vi "nRF24 communication.vi"(8 "error in (no error)":errorcluster) -> (0 "error out":errorcluster)   [LabVIEW 2016]
uses:
  Typedef/Remote Control Cluster.ctl
  Typedef/INS Data.ctl
  Shared resoruces/gear.vi
  Shared resoruces/ODrive State and Info.vi
  Shared resoruces/Navigation Variables.vi
  Shared resoruces/Shared resources RT.lvlib
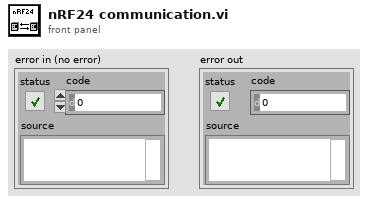
[diagram p1: front panel]
types:
  T1 = typedef "Semaphore RefNum" = refnum<k1>
  T2 = typedef "INS Data.ctl" = cluster{"Yaw":sgl, "Pitch":sgl, "Roll":sgl, "Lat":dbl, "Long":dbl, "Alt":dbl, "North":dbl, "East":dbl, "Down":dbl, "PosU":dbl, "VelU":dbl}
  T3 = typedef "Remote Control Cluster.ctl" = cluster{"Pot1":u16, "Pot2":u16, "Pot3":u16, "Pot4":u16, "Switch1":cluster{"L":bool, "H":bool}, "Switch2":cluster{"L":bool, "H":bool}, "Switch3":cluster{"L":bool, "H":bool}}
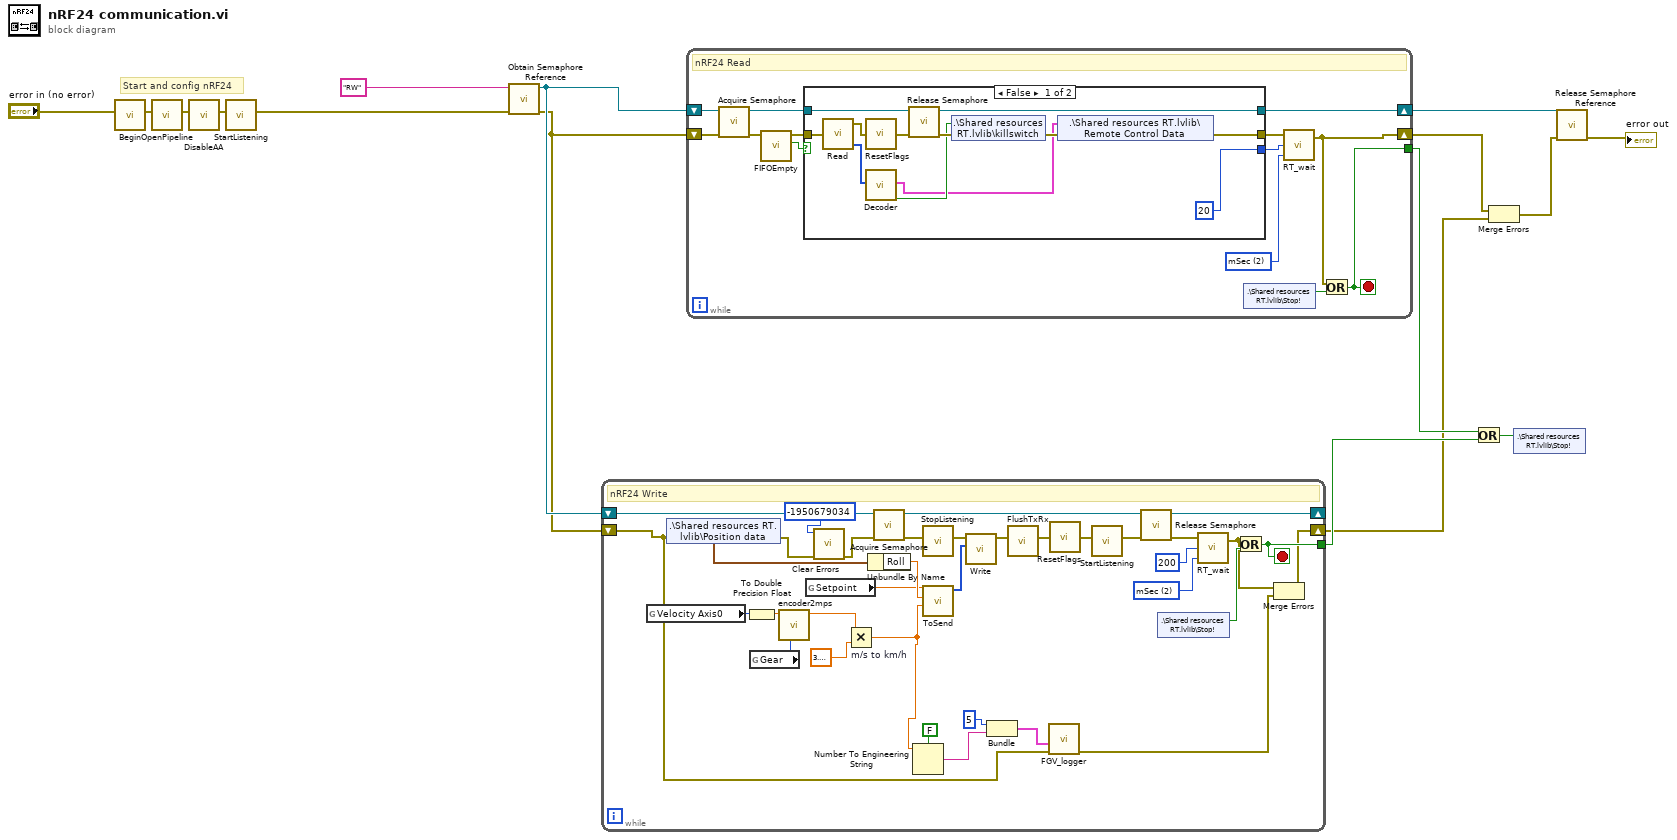
[diagram p0: block diagram]
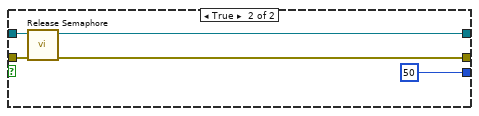
[diagram p2: hidden frame]
diagram:
  # "Start and config nRF24"
  n1 = call "Begin.vi"("error in (no error)"="error in (no error)") -> ("error out"=w2:errorcluster)  [unwired: 10 in]
  n2 = call "OpenPipeline.vi"("error in (no error)"=w2) -> ("error out"=w3:errorcluster)  [unwired: 10 in]
  n3 = call "DisableAA.vi"("error in (no error)"=w3) -> ("error out"=w4:errorcluster)  [unwired: 10 in]
  n4 = call "StartListening.vi"("error in (no error)"=w4) -> ("error out"=w5:errorcluster)  [unwired: 10 in]
  n5 = call <vilib>:"Obtain Semaphore Reference.vi"("error in (no error)"=w5, "name (unnamed)"="RW") -> ("error out"=w7:errorcluster, "semaphore"=w8:T1)  [unwired: 3 in, 1 out]
  n6 = while {
    shift-right: [w45] -> _
    shift-left: w8 -> [w51]
    shift-right: [w28] -> w10
    shift-left: w7 -> [w30]
    tunnel: [w36] -> w14
    stop <- w36 stop-if-true
    w42 = u16 2 items=["Ticks", "uSec", "mSec"] ("Counter Units")
    # "nRF24 Write"
    n7 = global read "ODrive State and Info.vi" "Velocity Axis0"() -> (w19:i16)
    n8 = shared-variable ".\\Shared resources RT.lvlib\\Position data"(error in=w30) -> (w35:T2, error out=w26:errorcluster)
    n9 = To Double Precision Float(number=w19) -> (double precision float=w18:dbl)
    n10 = global read "gear.vi" "Gear"() -> (w20:enum16{"7", "6", "5", "4", "3", "2", "1"})
    n11 = call "encoder2mps.vi"("Gear"=w20, "encoderSpeed"=w18) -> ("realVelocity"=w23:dbl)  [unwired: 9 in]
    n12 = global read "Navigation Variables.vi" "Setpoint"() -> (w17:dbl)
    n13 = call <vilib>:"Clear Errors.vi"("error in (no error)"=w26, "specific error code to clear (0: all)"=-1950679034) -> ("error out"=w25:errorcluster)  [unwired: 4 in, 1 out]
    n14 = Multiply "m/s to km/h"(x=w23, y=sgl 3.6) -> (x*y=w21:dbl)
    n15 = Unbundle By Name(w35) -> ("Roll"=w41:sgl)
    n16 = call <vilib>:"Acquire Semaphore.vi"("error in (no error)"=w25, "semaphore"=w51) -> ("error out"=w50:errorcluster, "semaphore out"=w46:T1)  [unwired: 3 in, 1 out]
    n17 = Number To Engineering String(1:FALSE ("use system decimal point (T)"), 4:w21) -> (0:w31:string)  [unwired: 2 in]
    n18 = call "StopListening.vi"("error in (no error)"=w50) -> ("error out"=w40:errorcluster)  [unwired: 10 in]
    n19 = call "ToSend.vi"("velocity"=w21, "leanAngel"=w41, "setpoint"=w17) -> ("data2nRF24"=w38:u8[])  [unwired: 8 in]
    n20 = call "Write.vi"("Input"=w38, "error in (no error)"=w40) -> ("error out"=w39:errorcluster)  [unwired: 8 in, 1 out]
    n21 = Bundle(5, w31) -> (w33:cluster{i32, string})  [unwired: 1 in]
    n22 = call "FlushTxRx.vi"("error in (no error)"=w39) -> ("error out"=w49:errorcluster)  [unwired: 10 in]
    n23 = call "FGV_logger.vi"("error in"=w30, 9:w33) -> ("error out"=w27:errorcluster)  [unwired: 9 in]
    n24 = call "ResetFlags.vi"("error in (no error)"=w49) -> ("error out"=w48:errorcluster)
    n25 = call "StartListening.vi"("error in (no error)"=w48) -> ("error out"=w47:errorcluster)  [unwired: 10 in]
    n26 = call <vilib>:"Release Semaphore.vi"("error in (no error)"=w47, "semaphore"=w46) -> ("error out"=w44:errorcluster, "semaphore out"=w45:T1)  [unwired: 4 in]
    n27 = shared-variable ".\\Shared resources RT.lvlib\\Stop!"() -> (w37:bool)  [unwired: 1 in, 1 out]
    n28 = call "RT_wait.vi"("Counter Units"=w42, "Count(mSec)"=u32 200 ("Count(uSec)"), "error in (no error)"=w44) -> ("error out"=w29:errorcluster)  [unwired: 1 in, 1 out]
    n29 = Or(x=w29, y=w37) -> (x .or. y?=w36:bool)
    n30 = Merge Errors(w29, w27) -> (w28:errorcluster)
  }
  n31 = while {
    shift-right: [w59] -> w9
    shift-left: w8 -> [w64]
    shift-right: [w53] -> w11
    shift-left: w7 -> [w63]
    tunnel: [w52] -> w15
    stop <- w52 stop-if-true
    w56 = u16 2 items=["Ticks", "uSec", "mSec"] ("Counter Units")
    # "nRF24 Read"
    n32 = call <vilib>:"Acquire Semaphore.vi"("error in (no error)"=w63, "semaphore"=w64) -> ("error out"=w62:errorcluster, "semaphore out"=w60:T1)  [unwired: 3 in, 1 out]
    n33 = call "FIFOEmpty.vi"("error in (no error)"=w62) -> ("RX_EMPTY"=w58:bool, "error out"=w61:errorcluster)  [unwired: 9 in]
    n34 = case shown="False" w58 {
      tunnel: w61 -> [w76 w81]
      tunnel: w60 -> [w73 w80]
      tunnel: [w65 w78] -> w57
      tunnel: [w72 w79] -> w59
      tunnel: [u32 20 ("Count(uSec)") u32 50 ("Count(uSec)")] -> w55
      frame False {
        n35 = call "Read.vi"("error in (no error)"=w76) -> ("error out"=w75:errorcluster, "Data frame"=w71:u16[])  [unwired: 1 out]
        n36 = call "ResetFlags.vi"("error in (no error)"=w75) -> ("error out"=w74:errorcluster)
        n37 = call "Decoder.vi"("Data frame"=w71) -> ("output cluster"=w66:T3, "Kill Switch"=w68:bool)  [unwired: 17 in]
        n38 = call <vilib>:"Release Semaphore.vi"("error in (no error)"=w74, "semaphore"=w73) -> ("error out"=w69:errorcluster, "semaphore out"=w72:T1)  [unwired: 4 in]
        n39 = shared-variable ".\\Shared resources RT.lvlib\\killswitch"(w68, error in=w69) -> (error out=w67:errorcluster)
        n40 = shared-variable ".\\Shared resources RT.lvlib\\Remote Control Data"(w66, error in=w67) -> (error out=w65:errorcluster)
      }
      frame True {
        n41 = call <vilib>:"Release Semaphore.vi"("error in (no error)"=w81, "semaphore"=w80) -> ("error out"=w78:errorcluster, "semaphore out"=w79:T1)  [unwired: 4 in]
      }
    }
    n42 = shared-variable ".\\Shared resources RT.lvlib\\Stop!"() -> (w54:bool)  [unwired: 1 in, 1 out]
    n43 = call "RT_wait.vi"("Counter Units"=w56, "Count(mSec)"=w55, "error in (no error)"=w57) -> ("error out"=w53:errorcluster)  [unwired: 1 in, 1 out]
    n44 = Or(x=w53, y=w54) -> (x .or. y?=w52:bool)
  }
  n45 = Or(x=w15, y=w14) -> (x .or. y?=w13:bool)
  n46 = Merge Errors(w11, w10) -> (w12:errorcluster)
  n47 = shared-variable ".\\Shared resources RT.lvlib\\Stop!"(w13) -> ()  [unwired: 1 in, 1 out]
  n48 = call <vilib>:"Release Semaphore Reference.vi"("error in (no error)"=w12, "semaphore"=w9) -> ("error out"=→"error out":errorcluster)  [unwired: 8 in, 1 out]
